vi "save_raster_image.vi"(8 "error in (no error)":errorcluster, 11 "scan_2d_hdf5_log in":refnum<class "scan_2d_hdf5_log.lvclass">) -> (0 "error out":errorcluster, 3 "scan_2d_hdf5_log out":refnum<class "scan_2d_hdf5_log.lvclass">)   [LabVIEW 2015, in "scan_2d_hdf5_log.lvclass"]
uses:
  scan_2d_hdf5_log.lvclass
  scan_2d_hdf5_log.lvclass/scan_2d_hdf5_log.ctl
  <vilib>/Utility/miscctls.llb/LVRectTypeDef.ctl
  <vilib>/UPVI/lvhdf5/group.llb/H5G_obj_t.ctl
  <vilib>/UPVI/lvhdf5/dataset.llb/LVH5D Operation.ctl
  <vilib>/UPVI/lvhdf5/utility.llb/Select HDF5 Dialog.vi
  <vilib>/UPVI/lvhdf5/utility.llb/Select HDF5 Dialog (Object Only).vi
  <vilib>/UPVI/lvhdf5/dataset.llb/Simple H5Dwrite (Variant).vi
  <vilib>/UPVI/lvhdf5/dataset.llb/Simple H5Dwrite.xnode
  <vilib>/UPVI/lvhdf5/library.llb/HDF5 Ref.ctl
  <vilib>/UPVI/lvhdf5/file.llb/H5Fclose.vi
  <vilib>/UPVI/lvhdf5/identifier.llb/Not an HDF5 Refnum Constant.vi
  <vilib>/Utility/error.llb/Error Cluster From Error Code.vi
  <vilib>/UPVI/lvhdf5/dataset.llb/OpenCreateReplace Dataset by Element Type.vi
  <vilib>/UPVI/lvhdf5/dataspace.llb/H5Sselect_hyperslab.vi
  <vilib>/UPVI/lvhdf5/dataset.llb/H5Dwrite (Variant).vi
  <vilib>/UPVI/lvhdf5/dataset.llb/H5Dget_space.vi
  <vilib>/UPVI/lvhdf5/attribute.llb/private/LVH5AwriteWDTAttrs.vi
  <vilib>/UPVI/lvhdf5/dataspace.llb/H5Sclose.vi
  <vilib>/UPVI/lvhdf5/file.llb/OpenCreateReplace HDF5 File.vi
  <vilib>/UPVI/lvhdf5/file.llb/LVH5F Operation.ctl
  <vilib>/UPVI/lvhdf5/utility.llb/Select HDF5 Dialog (File and Object).vi
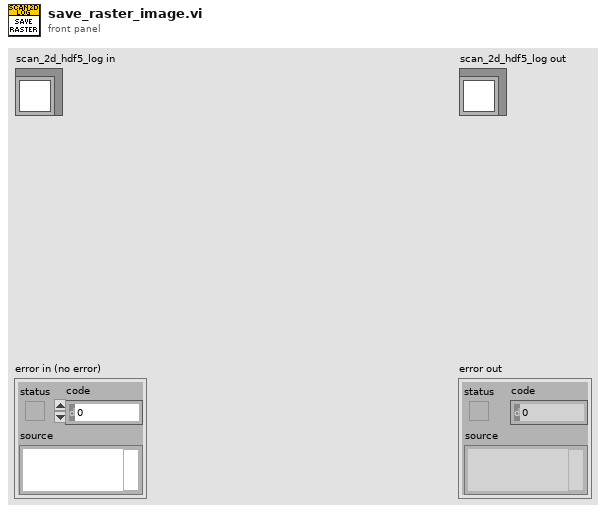
[diagram p1: front panel]
types:
  T1 = typedef "LVRectTypeDef.ctl" = cluster{"Left":i16, "Top":i16, "Right":i16, "Bottom":i16}
  T2 = cluster{"Behavior":enum32{"Invalid", "Default", "Floating", "Floating/Auto-Hide", "Modal"}, "Position":T1, "Center":bool, "Title":string}
  T3 = typedef "LVH5F Operation.ctl" = enum16{"open", "open or create", "create or replace", "create or replace (with confirmation)", "create", "open (read only)"}
  T4 = typedef "LVH5D Operation.ctl" = enum16{"open", "replace", "create", "open or create", "create or replace", "create or replace with confirmation"}
  T5 = typedef "H5G_obj_t.ctl" = i32
  T6 = cluster{"Object Types (any)":T5[], "Object Pattern":string}
  T7 = typedef "HDF5 Ref.ctl" = refnum<k1>
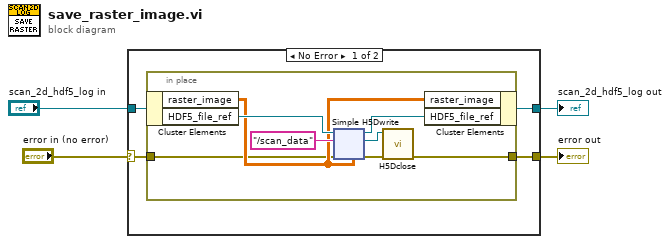
[diagram p0: block diagram]
diagram:
  n1 = case shown="No Error" "error in (no error)" {
    selector: "error in (no error)" -> [w7 w220]
    tunnel: [w8 w220] -> w3
    tunnel: [w5 w219] -> w1
    tunnel: "scan_2d_hdf5_log in" -> [w6 w219]
    frame No Error {
      n2 = in-place {
        in-place-border: [w10] -> w8
        in-place-border: w7 -> [w9]
        n3 = in-place-cluster #1(w6) -> ("raster_image"=w11:dbl[][], "HDF5_file_ref"=w16:T7)
        n4 = xnode "Simple H5Dwrite"("Dataset Path"="/scan_data", "error in (no error)"=w9, "HDF5 Path or Ref"=w16, "Data"=w11) -> ("HDF5 Dataset Ref out"=w14:T7, "HDF5 Ref out"=w12:T7, "error out"=w13:errorcluster)  [unwired: 4 in]
        n5 = call <vilib>:"H5Dclose.vi"("error in (no error)"=w13, "HDF5 Dataset Ref"=w14) -> ("error out"=w10:errorcluster)  [unwired: 7 in]
        n6 = in-place-cluster #1("raster_image"=w11, "HDF5_file_ref"=w12) -> (w5:refnum<class "scan_2d_hdf5_log.lvclass">)
      }
    }
    frame Error {
    }
  }
  "error out" <- w3
  "scan_2d_hdf5_log out" <- w1
